vi "Main.vi"() -> ()   [LabVIEW 2018, in "Application.lvlib"]
doc: "This VI is the main application VI in the Delacor QMH project template. This application VI is implemented as a simple state machine, which communicates with two different Delacor QMH modules.\n_____\nBased on Delacor QMH Project Template 4.1.0.59."
uses:
  Application.lvlib
  Application Data--cluster.ctl
  State--enum.ctl
  Data.vi
  MSG.vi
  MQTT_Singleton/MQTT_Singleton.lvlib
  MQTT Messages.lvlib
panel:
  in  "Temp":dbl(slide) scale=0.0..10.0
  in  "Current":dbl(slide) scale=0.0..10.0
  in  "Voltage":dbl(slide) scale=0.0..10.0
  out "Connection OK?":bool
  in  "Subscribe Topic":string
  in  "ClientID":string
  in  "Broker IP":string="test.mosquitto.org"
  in  "Subscribe":bool
  in  "Connect":bool
  in  "MSG":string="START TEST CMD Recieved"
  in  "Send MSG":bool
  out "Data Table":string[][](table)=[["Description", "Test Bay 1"], ["Version", "0.1"], ["", ""], ["", ""], ["", ""]]
  out "RX Message":string
  out "RX Topic":string
  out "version":string
  in  "Hide MQTT_Singleton Module":bool
  in  "Show MQTT_Singleton Module":bool
  in  "Stop MQTT_Singleton Module":bool
  in  "Start MQTT_Singleton Module":bool
  out "MQTT_Singleton Running?":bool
  out "Status":string
  # "1. Start the MQTT module\n2. Connect to the broker. On successful connection the application will send data every 2 seconds"
  # "1"
  # "2"
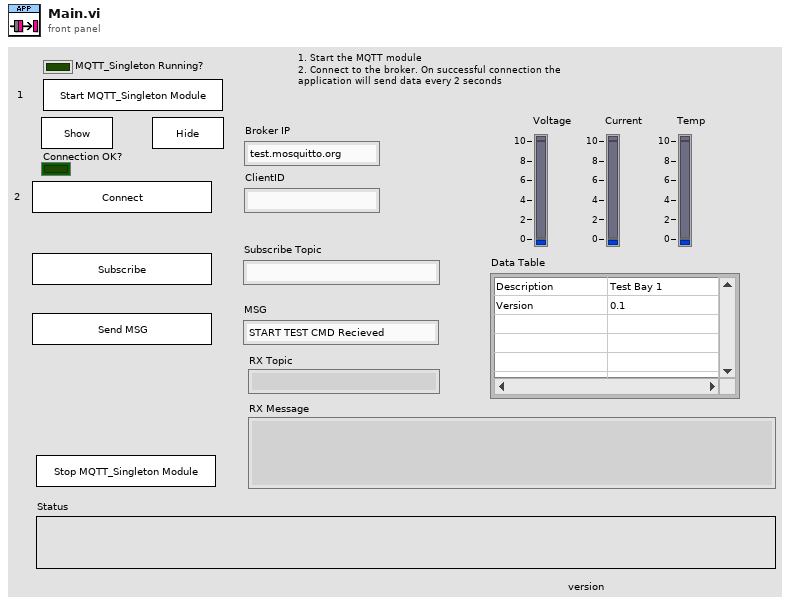
[diagram p1: front panel]
types:
  T1 = typedef "Application.lvlib/State--enum.ctl" = enum16{"Initialize", "Initialize Panel", "UI Interlocks", "Update Status", "Wait for Event", "Exit"}
  T2 = typedef "Application.lvlib/Application Data--cluster.ctl" = cluster{"Status":string, "Singleton Controls":refnum<vi>[], "Connection OK?":bool}
  T3 = typedef "MQTT_Singleton.lvlib/Broadcast Events--cluster.ctl" = cluster{"Module Did Init":refnum<user-event>, "Status Updated":refnum<user-event>, "Error Reported":refnum<user-event>, "Module Did Stop":refnum<user-event>, "Update Module Execution Status":refnum<user-event>, "RX":refnum<user-event>, "Connection Status":refnum<user-event>}
  T4 = enum8{"Enabled", "Disabled", "Disabled and Grayed Out"}
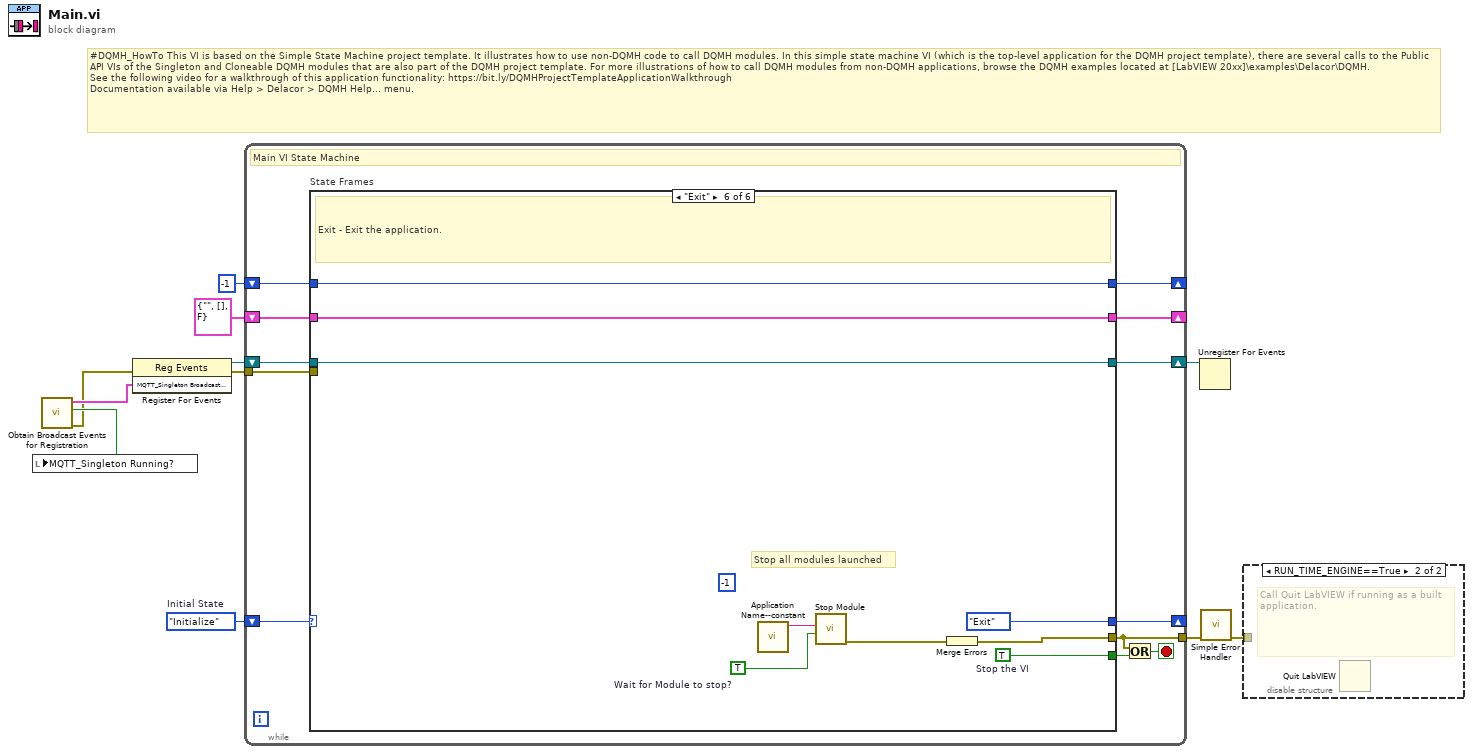
[diagram p0: block diagram]
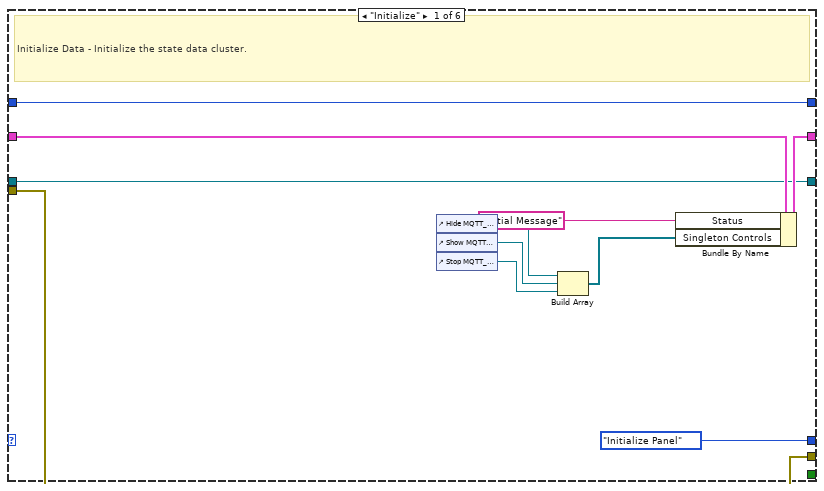
[diagram p2: hidden frame]
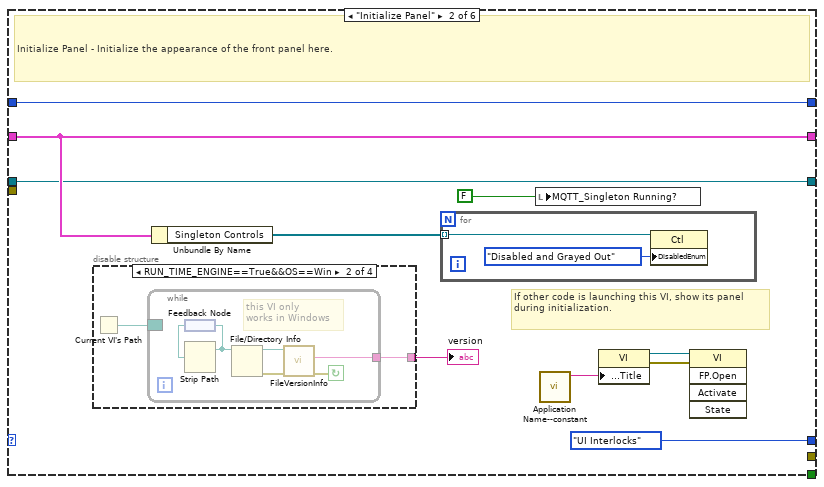
[diagram p3: hidden frame]
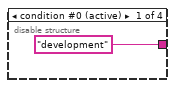
[diagram p4: hidden frame]
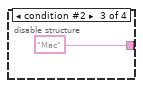
[diagram p5: hidden frame]
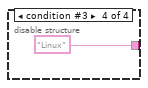
[diagram p6: hidden frame]
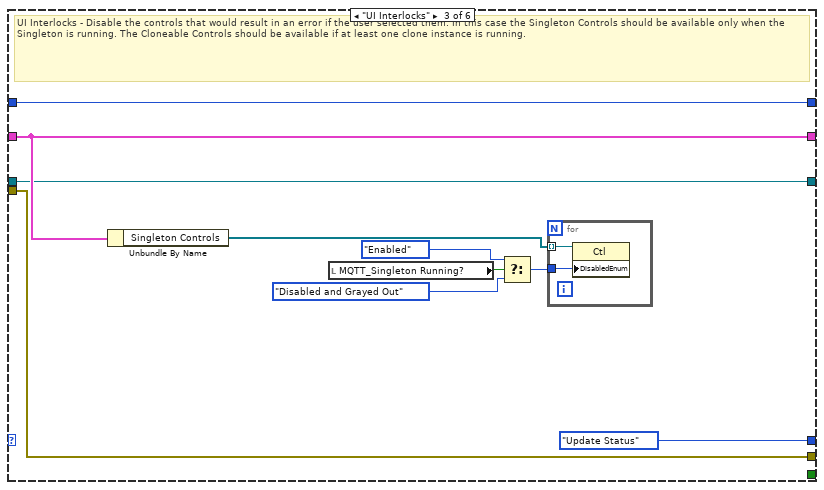
[diagram p7: hidden frame]
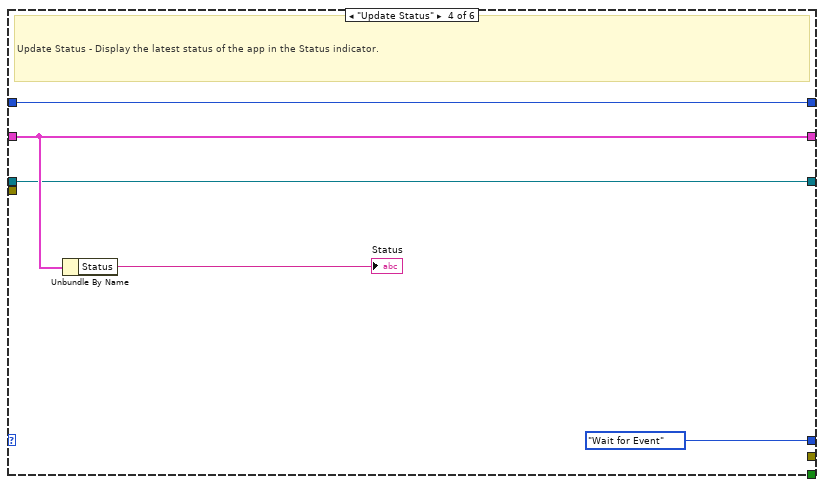
[diagram p8: hidden frame]
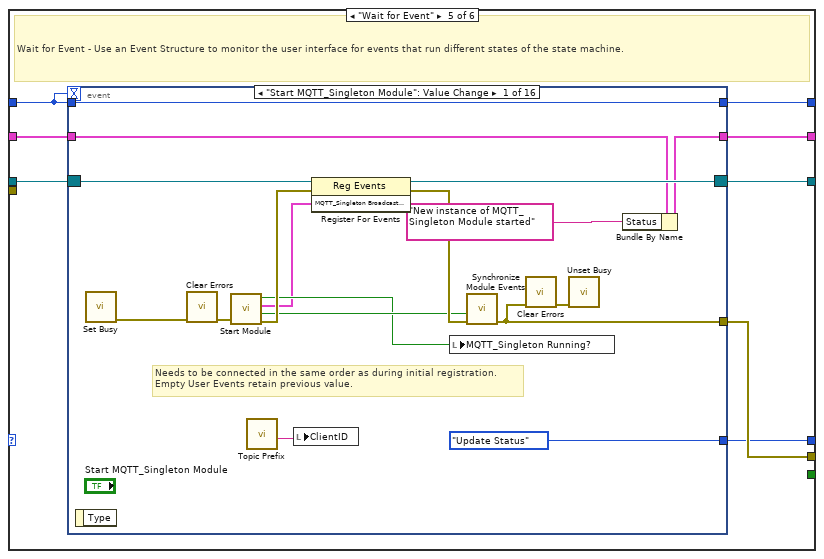
[diagram p9: hidden frame]
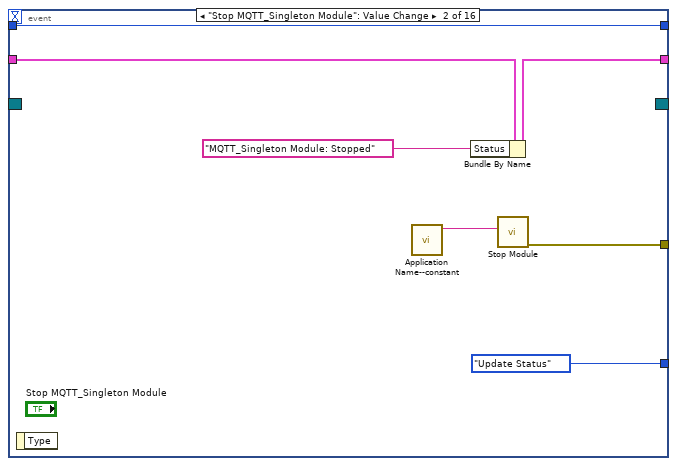
[diagram p10: hidden frame]
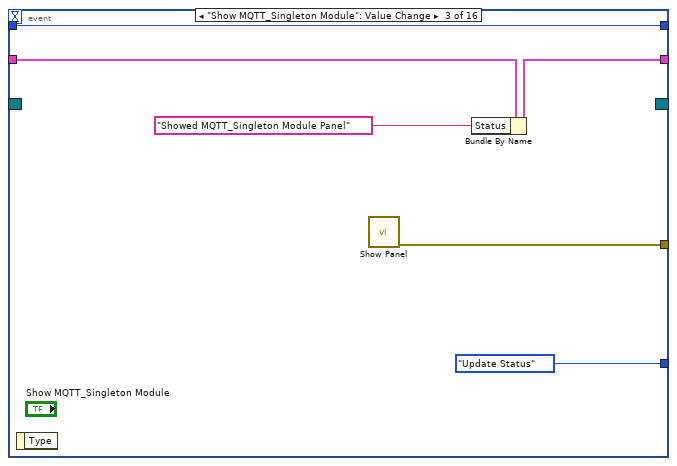
[diagram p11: hidden frame]
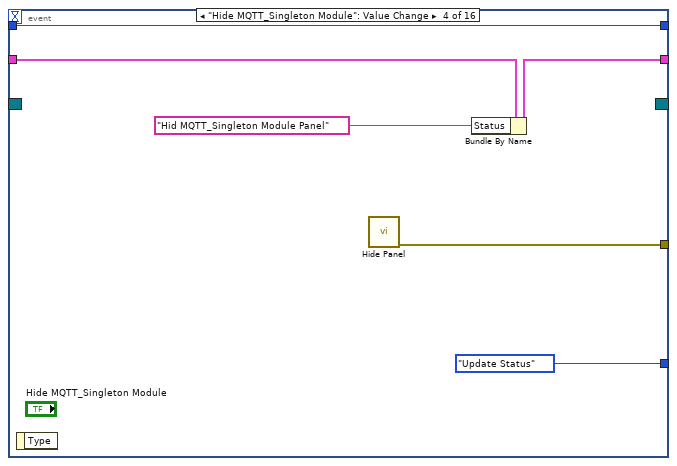
[diagram p12: hidden frame]
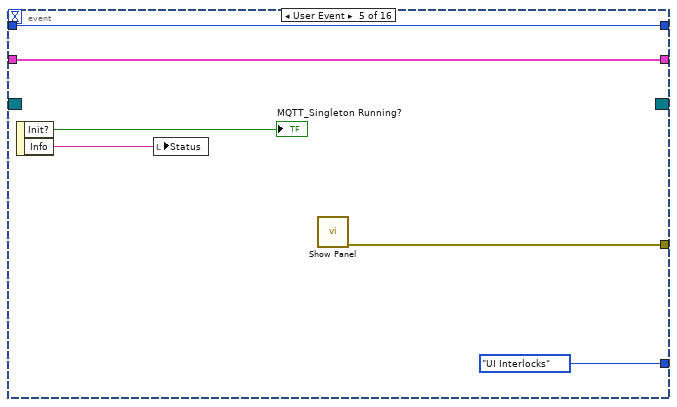
[diagram p13: hidden frame]
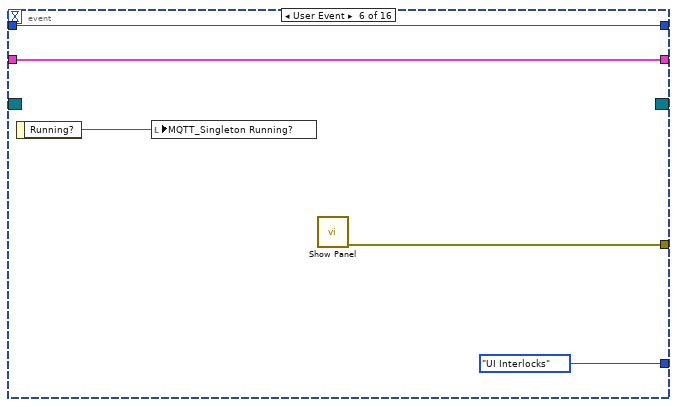
[diagram p14: hidden frame]
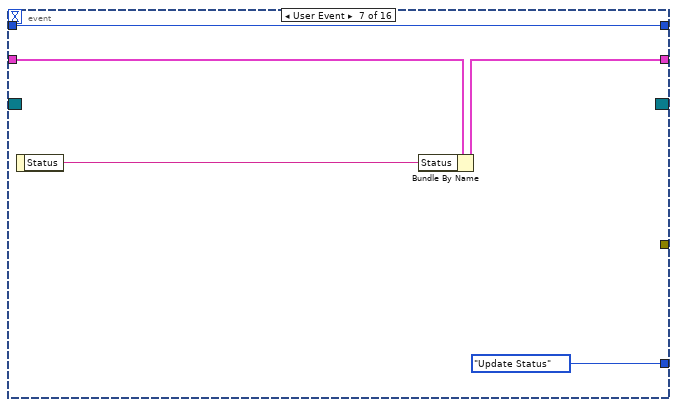
[diagram p15: hidden frame]
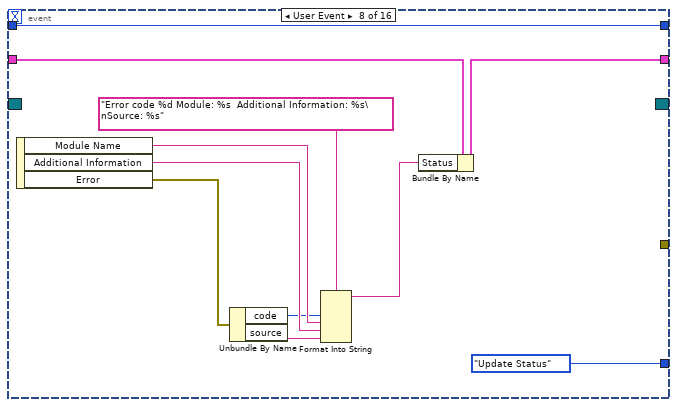
[diagram p16: hidden frame]
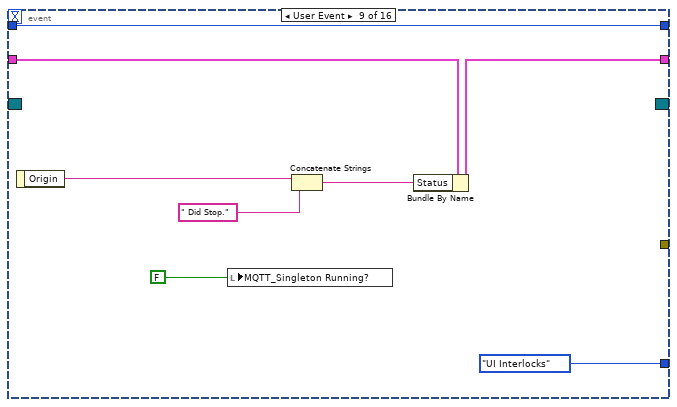
[diagram p17: hidden frame]
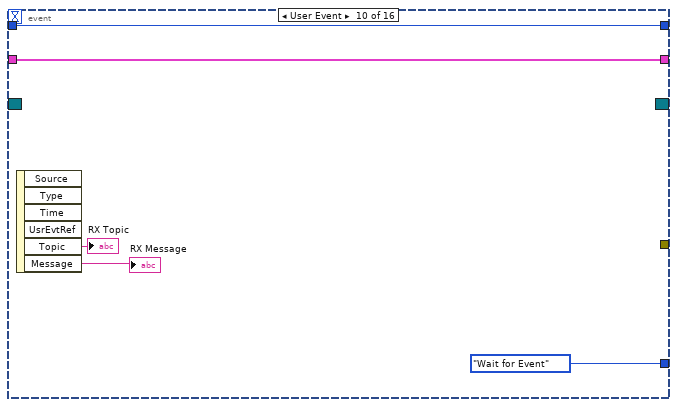
[diagram p18: hidden frame]
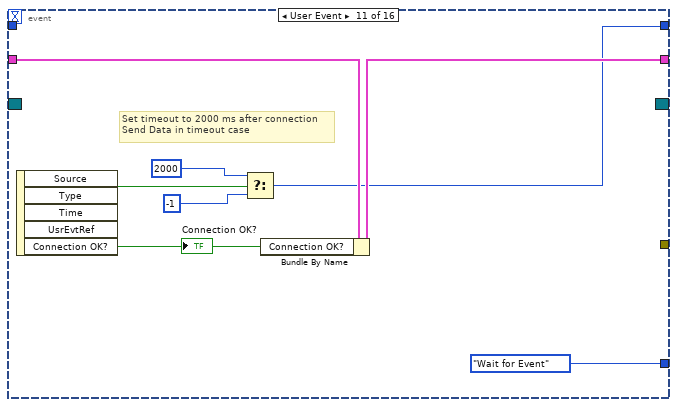
[diagram p19: hidden frame]
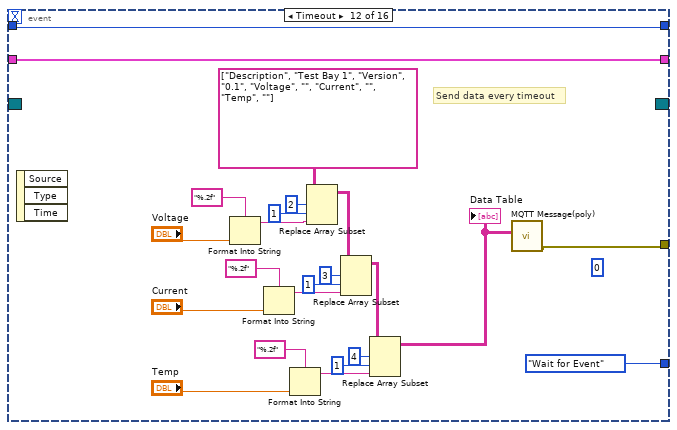
[diagram p20: hidden frame]
diagram:
  w6 = State--enum."Initialize"  # Initial State
  # "#DQMH_HowTo This VI is based on the Simple State Machine project template. It illustrates how to use non-DQMH code to call DQMH modules. In this simple state machine VI (which is the top-level application for the DQMH project template), there are several calls to the Public API VIs of the Singleton and Cloneable DQMH modules that are also part of the DQMH project template. For more illustrations of how to call DQMH modules from non-DQMH applications, browse the DQMH examples located at [LabVIEW 20xx]\\examples\\Delacor\\DQMH.\nSee the following video for a walkthrough of this application functionality: https://bit.ly/DQMHProjectTemplateApplicationWalkthrough\nDocumentation available via Help > Delacor > DQMH Help... menu."
  n1 = call "Obtain Broadcast Events for Registration.vi"() -> ("error out"=w2:errorcluster, "Already running?"=w3:bool, "MQTT_Singleton Broadcast Events"=w7:T3)  [unwired: 9 in]
  n2 = local write "MQTT_Singleton Running?"(w3) -> ()
  n3 = register-events(error in=w2, w7) -> (reference out=w5:refnum<event-registration>, error out=w9:errorcluster)  [unwired: 1 in]
  n4 = while {
    shift-right: [w20] -> _
    shift-left: T2 {"Status"="", "Singleton Controls"=[], "Connection OK?"=FALSE} ("Data Cluster") -> [w21]
    tunnel: [w23] -> w11
    shift-right: [w16] -> _
    shift-left: w6 -> [w18]
    shift-right: [w14] -> w4
    shift-left: w5 -> [w15]
    tunnel: w9 -> [w22]
    shift-right: [w12] -> _
    shift-left: -1 -> [w13]
    stop <- w17 stop-if-true
    # "Main VI State Machine"
    n5 = case "State Frames" shown="\"Exit\"" w18 {
      tunnel: [w34 _ w59 _ w82 w216] -> w23
      tunnel: w21 -> [w33 w42 w62 w74 w79 w214]
      tunnel: [w32 w42 w62 w74 w78 w214] -> w20
      tunnel: [_ _ _ _ _ w213] -> w19
      tunnel: [State--enum."Initialize Panel" ("State") State--enum."UI Interlocks" ("State") State--enum."Update Status" ("State") State--enum."Wait for Event" ("State") w77 State--enum."Exit" ("State")] -> w16
      tunnel: w15 -> [w25 w39 w60 w71 w81 w211]
      tunnel: [w25 w39 w60 w71 w80 w211] -> w14
      tunnel: w22 -> [w34 _ w59 _ _ _]
      tunnel: w13 -> [w24 w35 w58 w70 w75 w208]
      tunnel: [w24 w35 w58 w70 w76 w208] -> w12
      frame "Initialize" {
        # "Initialize Data - Initialize the state data cluster."
        n6 = control-ref of="Hide MQTT_Singleton Module"() -> (w30:refnum<vi>)
        n7 = control-ref of="Show MQTT_Singleton Module"() -> (w29:refnum<vi>)
        n8 = control-ref of="Stop MQTT_Singleton Module"() -> (w28:refnum<vi>)
        n9 = Build Array(w30, w29, w28) -> (w27:refnum<vi>[])
        n10 = Bundle By Name(cluster=w33, "Status"="Initial Message" ("Initial Message"), "Singleton Controls"=w27) -> (w32:T2)
      }
      frame "Initialize Panel" {
        # "If other code is launching this VI, show its panel during initialization."
        # "Initialize Panel - Initialize the appearance of the front panel here."
        n11 = disable-structure "Conditional Disable Structure" shown="RUN_TIME_ENGINE==True&&OS==Win" {
          disable-tunnel: ["development" w46 "Mac" "Linux"] -> w38
          frame condition #0 (active) {
          }
          frame condition #1 {
            n12 = Current VI's Path() -> (path=w47:path)
            n13 = while {
              border: w47 -> [_]
              tunnel: [w48] -> w46
              stop <- w52 continue-if-true
              # "this VI only \nworks in Windows"
              n14 = feedback #1() -> (w51:path)
              n15 = Strip Path(path=w51) -> (stripped path=w50:path)  [unwired: 1 out]
              n16 = feedback-in #1(w50) -> ()
              n17 = File/Directory Info(path=w50) -> (path out=w49:path, error out=w53:errorcluster)  [unwired: 1 in, 5 out]
              n18 = call <vilib>:"FileVersionInfo.vi"("error in (no error)"=w53, "Application Path in"=w49) -> ("error out"=w52:errorcluster, "File Version Info"=w48:string)  [unwired: 6 in, 2 out]
            }
          }
          frame condition #2 {
          }
          frame condition #3 {
          }
        }
        "version" <- w38
        n19 = Unbundle By Name(w42) -> ("Singleton Controls"=w41:refnum<vi>[])
        n20 = for {
          tunnel: w41 -> [w57] mode=indexing
          n21 = property on="Property Node" class="Ctl"(reference=w57, "DisabledEnum"=T4."Disabled and Grayed Out" ("Disabled")) -> ()  [unwired: 1 in, 2 out]
        }
        n22 = local write "MQTT_Singleton Running?"(FALSE ("My Singleton Module Init?")) -> ()
        n23 = call "Application Name--constant.vi"() -> ("Application Name"=w37:string)  [unwired: 11 in]
        n24 = property on="Property Node" class="VI"("Front Panel.Title"=w37) -> (reference out=w36:refnum<vi>, error out=w44:errorcluster)  [unwired: 2 in]
        n25 = invoke class="VI" method="FP.Open"(reference=w36, error in=w44) -> ()  [unwired: 3 in, 5 out]
      }
      frame "UI Interlocks" {
        # "UI Interlocks - Disable the controls that would result in an error if the user selected them. In this case the Singleton Controls should be available only when the Singleton is running. The Cloneable Controls should be available if at least one clone instance is running."
        n26 = Unbundle By Name(w62) -> ("Singleton Controls"=w64:refnum<vi>[])
        n27 = local read "MQTT_Singleton Running?"() -> (w63:bool)
        n28 = Select(t=T4."Enabled" ("Disabled"), s=w63, f=T4."Disabled and Grayed Out" ("Disabled")) -> (s? t:f=w65:T4)
        n29 = for {
          tunnel: w64 -> [w69] mode=indexing
          tunnel: w65 -> [w68]
          n30 = property on="Property Node" class="Ctl"(reference=w69, "DisabledEnum"=w68) -> ()  [unwired: 1 in, 2 out]
        }
      }
      frame "Update Status" {
        # "Update Status - Display the latest status of the app in the Status indicator."
        n31 = Unbundle By Name(w74) -> ("Status"=→"Status":string)
      }
      frame "Wait for Event" {
        # "Wait for Event - Use an Event Structure to monitor the user interface for events that run different states of the state machine."
        n32 = event shown="[0] \"Start MQTT_Singleton Module\": Value Change" {
          selector: w81 -> [w92 _ _ _ _ _ _ _ _ _ _ _ _ _ _ _]
          dyn-events: [w91 _ _ _ _ _ _ _ _ _ _ _ _ _ _ _] -> w80
          timeout: w75 -> [_ _ _ _ _ _ _ _ _ _ _ _ _ _ _ _]
          tunnel: [w99 w106 w112 w118 w124 w129 _ _ _ _ _ w186 _ w194 w201 _] -> w82
          tunnel: [w88 w102 w110 w116 w121 w128 w132 w143 w150 w158 w164 w185 w192 w198 w203 w206] -> w78
          tunnel: w79 -> [w89 w103 w111 w117 w121 w128 w133 w144 w151 w158 w165 w185 w192 w198 w203 w206]
          tunnel: [State--enum."Update Status" ("State") State--enum."Update Status" ("State") State--enum."Update Status" ("State") State--enum."Update Status" ("State") State--enum."UI Interlocks" ("State") State--enum."UI Interlocks" ("State") State--enum."Update Status" ("State") State--enum."Update Status" ("State") State--enum."UI Interlocks" ("State") State--enum."Wait for Event" ("State") State--enum."Wait for Event" ("State") State--enum."Wait for Event" ("State") State--enum."Wait for Event" ("State") State--enum."Wait for Event" ("State") State--enum."Wait for Event" ("State") State--enum."Exit" ("State")] -> w77
          tunnel: [w84 w100 w107 w113 w119 w125 w130 w135 w146 w154 w159 w188 w189 w193 w199 w204] -> w76
          tunnel: w75 -> [w84 w100 w107 w113 w119 w125 w130 w135 w146 w154 _ w188 w189 w193 w199 w204]
          event "Start MQTT_Singleton Module": Value Change {
            # "Needs to be connected in the same order as during initial registration.\nEmpty User Events retain previous value."
            n33 = event-data() -> ()  [unwired: 1 in, 1 out]
            n34 = call <vilib>:"Set Busy.vi"() -> ("error out"=w95:errorcluster)  [unwired: 10 in, 1 out]
            n35 = call <vilib>:"Clear Errors.vi"("error in (no error)"=w95) -> ("error out"=w96:errorcluster)  [unwired: 5 in, 1 out]
            n36 = call "Start Module.vi"("error in (no error)"=w96) -> ("error out"=w98:errorcluster, "Wait for Event Sync?"=w93:bool, "MQTT_Singleton Broadcast Events"=w85:T3, "Module Was Already Running?"=w86:bool)  [unwired: 7 in]
            n37 = call "Topic Prefix.vi"() -> ("SN"=w83:string)  [unwired: 10 in, 1 out]
            n38 = local write "ClientID"(w83) -> ()
            n39 = register-events(reference=w92, error in=w98, w85) -> (reference out=w91:refnum<event-registration>, error out=w97:errorcluster)
            n40 = local write "MQTT_Singleton Running?"(w86) -> ()
            n41 = call "Synchronize Module Events.vi"("error in (no error)"=w97, "Wait for Event Sync?"=w93) -> ("error out"=w99:errorcluster)  [unwired: 9 in]
            n42 = call <vilib>:"Clear Errors.vi"("error in (no error)"=w99) -> ("error out"=w94:errorcluster)  [unwired: 5 in, 1 out]
            n43 = call <vilib>:"Unset Busy.vi"("error in (no error)"=w94) -> ()  [unwired: 10 in, 1 out]
            n44 = Bundle By Name(cluster=w89, "Status"="New instance of MQTT_Singleton Module started") -> (w88:T2)
          }
          event "Stop MQTT_Singleton Module": Value Change {
            n45 = event-data() -> ()  [unwired: 1 in, 1 out]
            n46 = call "Application Name--constant.vi"() -> ("Application Name"=w104:string)  [unwired: 11 in]
            n47 = Bundle By Name(cluster=w103, "Status"="MQTT_Singleton Module: Stopped" ("Message")) -> (w102:T2)
            n48 = call "Stop Module.vi"("Origin"=w104) -> ("error out"=w106:errorcluster)  [unwired: 10 in]
          }
          event "Show MQTT_Singleton Module": Value Change {
            n49 = event-data() -> ()  [unwired: 1 in, 1 out]
            n50 = call "Show Panel.vi"() -> ("error out"=w112:errorcluster)  [unwired: 11 in]
            n51 = Bundle By Name(cluster=w111, "Status"="Showed MQTT_Singleton Module Panel" ("Message")) -> (w110:T2)
          }
          event "Hide MQTT_Singleton Module": Value Change {
            n52 = event-data() -> ()  [unwired: 1 in, 1 out]
            n53 = call "Hide Panel.vi"() -> ("error out"=w118:errorcluster)  [unwired: 11 in]
            n54 = Bundle By Name(cluster=w117, "Status"="Hid MQTT_Singleton Module Panel" ("Message")) -> (w116:T2)
          }
          event User Event {
            # "MQTT_Singleton Module has broadcast that it has been initialized"
            n55 = event-data() -> ("Init?"=→"MQTT_Singleton Running?":bool, "Info"=w123:string)  [unwired: 1 in]
            n56 = local write "Status"(w123) -> ()
            n57 = call "Show Panel.vi"() -> ("error out"=w124:errorcluster)  [unwired: 11 in]
          }
          event User Event {
            # "MQTT_Singleton Module has broadcast its execution status"
            n58 = event-data() -> ("Running?"=w126:bool)  [unwired: 1 in]
            n59 = local write "MQTT_Singleton Running?"(w126) -> ()
            n60 = call "Show Panel.vi"() -> ("error out"=w129:errorcluster)  [unwired: 11 in]
          }
          event User Event {
            # "MQTT_Singleton Module has broadcast its status"
            n61 = event-data() -> ("Status"=w134:string)  [unwired: 1 in]
            n62 = Bundle By Name(cluster=w133, "Status"=w134) -> (w132:T2)
          }
          event User Event {
            # "MQTT_Singleton Module had an error"
            n63 = event-data() -> ("Module Name"=w137:string, "Additional Information"=w141:string, "Error"=w145:errorcluster)  [unwired: 1 in]
            n64 = Unbundle By Name(w145) -> ("code"=w136:i32, "source"=w140:string)
            n65 = Format Into String(format string="Error code %d Module: %s  Additional Information: %s\nSource: %s", w136, w137, w141, w140) -> (resulting string=w138:string)  [unwired: 2 in, 1 out]
            n66 = Bundle By Name(cluster=w144, "Status"=w138) -> (w143:T2)
          }
          event User Event {
            n67 = event-data() -> ("Origin"=w148:string)  [unwired: 1 in]
            n68 = local write "MQTT_Singleton Running?"(FALSE ("My Singleton Module Init?")) -> ()
            n69 = Concatenate Strings(w148, " Did Stop.") -> (w147:string)
            n70 = Bundle By Name(cluster=w151, "Status"=w147) -> (w150:T2)
          }
          event User Event {
            n71 = event-data() -> ("Topic"=→"RX Topic":string, "Message"=→"RX Message":string)  [unwired: 1 in, 4 out]
          }
          event User Event {
            # "Set timeout to 2000 ms after connection\nSend Data in timeout case"
            n72 = event-data() -> ("Connection OK?"=w162:bool)  [unwired: 1 in, 4 out]
            "Connection OK?" <- w162
            n73 = Select(t=2000, s=w162, f=-1) -> (s? t:f=w159:i32)
            n74 = Bundle By Name(cluster=w165, "Connection OK?"=w162) -> (w164:T2)
          }
          event Timeout {
            (unwired) 0
            # "Send data every timeout"
            n75 = event-data() -> ()  [unwired: 1 in, 3 out]
            n76 = Format Into String(format string="%.2f", "Voltage") -> (resulting string=w180:string)  [unwired: 2 in, 1 out]
            n77 = Format Into String(format string="%.2f", "Current") -> (resulting string=w179:string)  [unwired: 2 in, 1 out]
            n78 = Format Into String(format string="%.2f", "Temp") -> (resulting string=w172:string)  [unwired: 2 in, 1 out]
            n79 = Replace Array Subset(array=string[][] [["Description", "Test Bay 1"], ["Version", "0.1"], ["Voltage", ""], ["Current", ""], ["Temp", ""]] ("Data Table"), new element=w180, index (row)=2, index (col)=1 ("disabled index (col)")) -> (w171:string[][])
            n80 = Replace Array Subset(array=w171, new element=w179, index (row)=3, index (col)=1 ("disabled index (col)")) -> (w170:string[][])
            n81 = Replace Array Subset(array=w170, new element=w172, index (row)=4, index (col)=1 ("disabled index (col)")) -> (w169:string[][])
            "Data Table" <- w169
            n82 = call-poly "MQTT Message(poly).vi"("Data"=w169) -> ("error out"=w186:errorcluster)  [unwired: 10 in]
          }
          event "Send MSG": Value Change {
            # "MSG topic is where you post status update messages similar to a system log.\nMessage posted here are sent to <SN>/MSG\nUse this topic to acknowledge commands, etc..."
            n83 = event-data() -> ()  [unwired: 1 in, 6 out]
            n84 = call-poly "MQTT Message(poly).vi"("Message"="MSG") -> ()  [unwired: 10 in, 1 out]
          }
          event "Connect": Value Change {
            n85 = event-data() -> ()  [unwired: 1 in, 6 out]
            n86 = call "Connect.vi"("ClientID"="ClientID", "Broker IP"="Broker IP") -> ("error out"=w194:errorcluster)  [unwired: 9 in]
          }
          event "Subscribe": Value Change {
            n87 = event-data() -> ()  [unwired: 1 in, 6 out]
            n88 = call "Subscribe.vi"("Topic"="Subscribe Topic") -> ("error out"=w201:errorcluster)  [unwired: 10 in]
          }
          event Panel Close? {
            # "Go to the 'Exit' state if the user tries to close the panel."
            n89 = event-data() -> ()  [unwired: 1 in, 1 out]
            n90 = event-data ("Event Filter Node")("Discard?"=TRUE) -> ()  [unwired: 1 in, 1 out]
          }
        }
      }
      frame "Exit" {
        w209 = TRUE  # Wait for Module to stop?
        (unwired) -1 ("Module ID")
        w213 = TRUE  # Stop the VI
        # "Stop all modules launched"
        # "Exit - Exit the application."
        n91 = call "Application Name--constant.vi"() -> ("Application Name"=w210:string)  [unwired: 11 in]
        n92 = call "Stop Module.vi"("Wait for Module to Stop? (F)"=w209, "Origin"=w210) -> ("error out"=w215:errorcluster)  [unwired: 9 in]
        n93 = Merge Errors(w215) -> (w216:errorcluster)
      }
    }
    n94 = Or(x=w23, y=w19) -> (x .or. y?=w17:bool)
  }
  n95 = Unregister For Events(event registration refnum=w4) -> ()  [unwired: 1 in, 1 out]
  n96 = call <vilib>:"Simple Error Handler.vi"("error in (no error)"=w11) -> ("error out"=w10:errorcluster)  [unwired: 4 in, 4 out]
  n97 = disable-structure "Conditional Disable Structure" shown="RUN_TIME_ENGINE==True" {
    disable-tunnel: w10 -> [_ _]
    frame condition #0 (active) {
    }
    frame condition #1 {
      # "Call Quit LabVIEW if running as a built application."
      n98 = Quit LabVIEW() -> ()  [unwired: 1 in]
    }
  }
